vi "PTSequencer.set modified data.vi"(0 "i ref in":refnum<vi>, 2 "CLASS.i attribute":T1, 5 "error in (no error)":errorcluster) -> (14 "i ref out":refnum<vi>, 19 "error out":errorcluster)   [LabVIEW 2014, in "PTSequencer.lvlib"]
uses:
  PTSequencer.lvlib
  PTSequencer.i attribute.ctl
  PTSequencer.mode.ctl
  PTSequencer.DIM service condition.ctl
  CSCore/CSSystem/CoreDefs/CoreDefs.rawDataType.ctl
  PTSequencer.step.ctl
  CSCore/CSObj/CSObj.lvlib
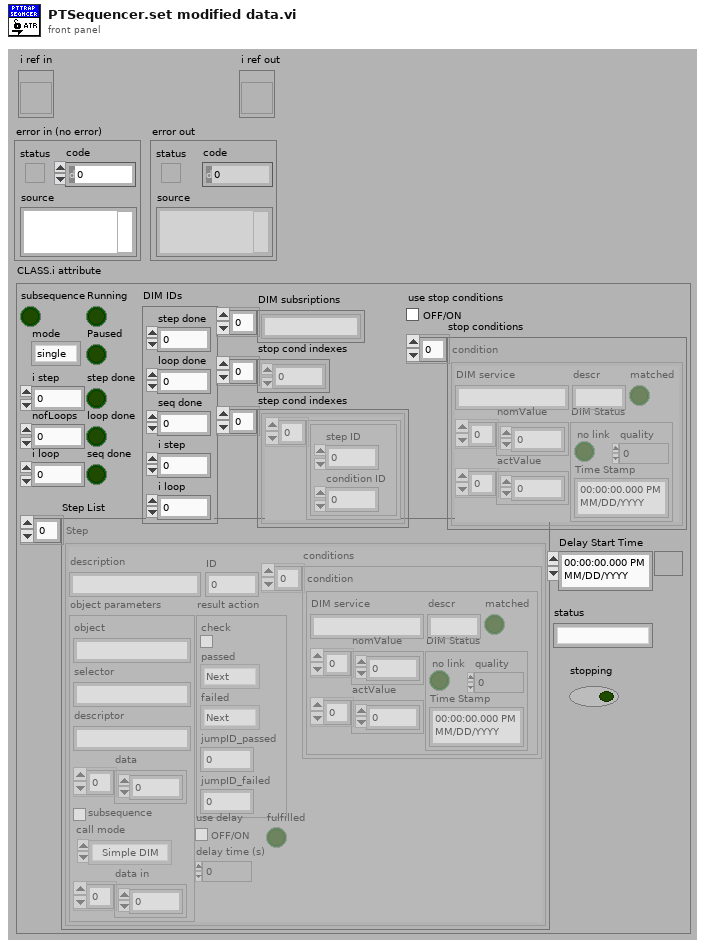
[diagram p1: front panel]
types:
  T1 = typedef "PTSequencer.lvlib/PTSequencer.i attribute.ctl" = cluster{"subsequence":bool, "mode":T2, "i step":i32, "nofLoops":i32, "i loop":i32, "Running":bool, "Paused":bool, "step done":bool, "loop done":bool, "seq done":bool, "DIM IDs":cluster{"step done":i32, "loop done":i32, "seq done":i32, "i step":i32, "i loop":i32}, "use stop conditions":bool, "stop conditions":T3[], "Step List":T5[], "DIM subsriptions":string[], "stop cond indexes":i32[], "step cond indexes":cluster{"step condition IDs":cluster{"step ID":i32, "condition ID":i32}[]}[], "Delay Start Time":timestamp, "status":string, "stopping":bool}
  T2 = typedef "PTSequencer.lvlib/PTSequencer.mode.ctl" = enum16{"single", "loop", "for loop"}
  T3 = typedef "PTSequencer.lvlib/PTSequencer.DIM service condition.ctl" = cluster{"DIM service":string, "descr":string, "nomValue":T4, "actValue":T4, "matched":bool, "DIM Status":cluster{"no link":bool, "quality":i32, "Time Stamp":timestamp}}
  T4 = typedef "CoreDefs.rawDataType.ctl" = i8[]
  T5 = typedef "PTSequencer.lvlib/PTSequencer.step.ctl" = cluster{"description":string, "object parameters":cluster{"object":string, "selector":string, "descriptor":string, "data":T4, "subsequence":bool, "call mode":enum16{"Simple DIM", "Synchronous"}, "data in":T4}, "result action":cluster{"check":bool, "passed":enum16{"Next", "Previous", "Repeat", "Jump"}, "failed":enum16{"Next", "Previous", "Repeat", "Jump"}, "jumpID_passed":i32, "jumpID_failed":i32}, "conditions":T3[], "fulfilled ":bool, "use delay":bool, "delay time (s)":dbl, "ID":i32}
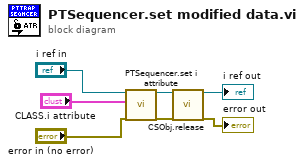
[diagram p0: block diagram]
diagram:
  n1 = call "PTSequencer.set i attribute.vi"("i ref in"="i ref in", "i attribute"="CLASS.i attribute", "error in (no error)"="error in (no error)") -> ("i ref out"=w5:refnum<vi>, "error out"=w4:errorcluster)  [unwired: 15 in]
  n2 = call "CSObj.release.vi"("i ref in"=w5, "error in (no error)"=w4) -> ("i ref out"=→"i ref out":refnum<vi>, "error out"=→"error out":errorcluster)  [unwired: 16 in]
